vi "get handler reference.vi"(11 "TLS HTTP server.lvclass":refnum<class "TLS HTTP server.lvclass">) -> (3 "VI Name":string)   [LabVIEW 2016, in "TLS HTTP server.lvclass"]
uses:
  TLS HTTP server.lvclass
  tls http connection handler.vi
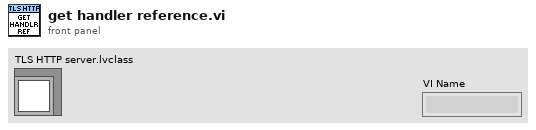
[diagram p1: front panel]
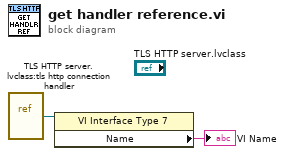
[diagram p0: block diagram]
diagram:
  n1 = vi-ref "TLS HTTP server.lvclass:tls http connection handler.vi"() -> (w1:refnum<vi>)
  n2 = property class="VI Interface Type 7"(reference=w1) -> ("Name"=→"VI Name":string)  [unwired: 1 in, 2 out]
